vi "GlobalSetGetHeidenhainParameters.vi"() -> ()   [LabVIEW 2013]
panel:
  in  "Z-Fokus":dbl
  in  "Clutch":bool
  in  "Up":bool
  in  "Down":bool
  in  "OutputParamers":T1
  out "ConfigurePosition":T2
  in  "Heidenhain Configure":T3
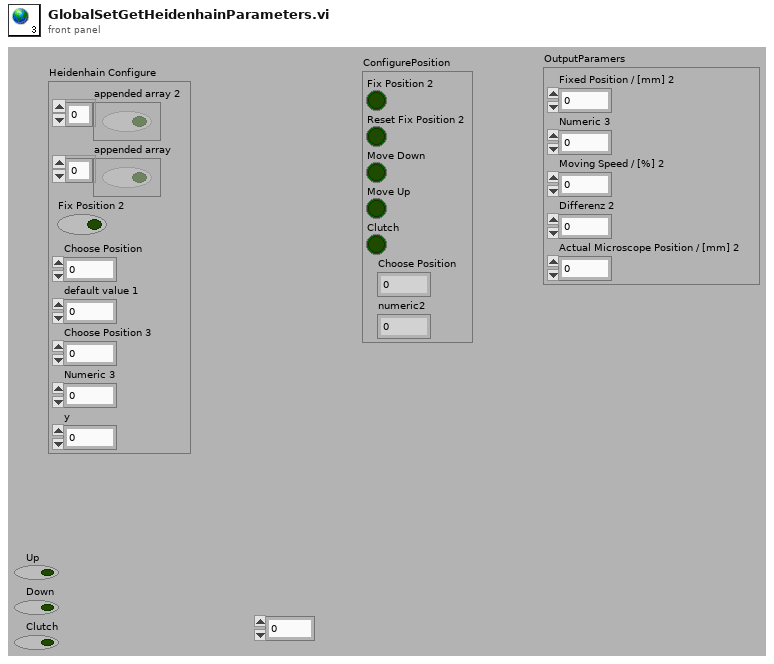
[diagram p1: front panel]
types:
  T1 = cluster{"Fixed Position / [mm] 2":dbl, "Numeric 3":dbl, "Moving Speed / [%] 2":i8, "Differenz 2":dbl, "Actual Microscope Position / [mm] 2":dbl}
  T2 = cluster{"Fix Position 2":bool, "Reset Fix Position 2":bool, "Move Down":bool, "Move Up":bool, "Clutch":bool, "Choose Position":dbl, "numeric2":dbl}
  T3 = cluster{"appended array 2":bool[], "appended array":bool[], "Fix Position 2":bool, "Choose Position":dbl, "default value 1":dbl, "Choose Position 3":dbl, "Numeric 3":i32, "y":i32}
diagram:
